vi "Valid data with Header (SubVI).vi"(10 "Header":string, 11 "Input data":string) -> (3 "Valid Data":string)   [LabVIEW 2021]
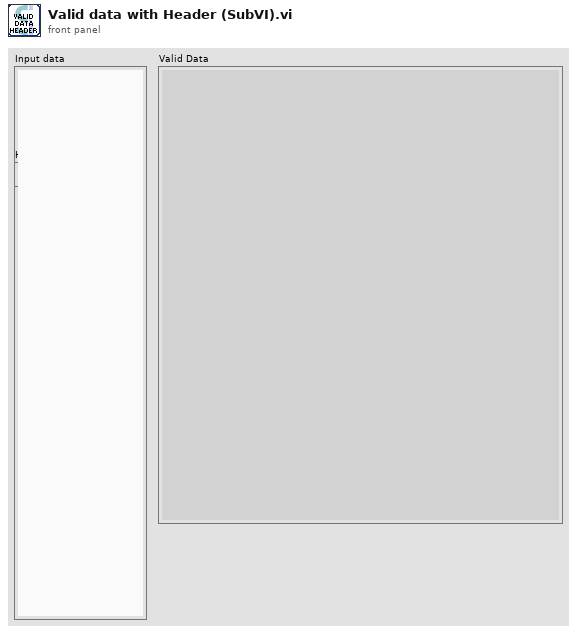
[diagram p1: front panel]
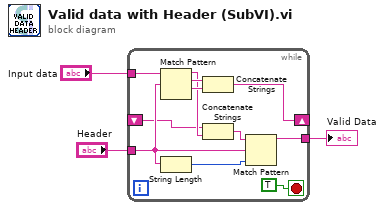
[diagram p0: block diagram]
diagram:
  n1 = while {
    tunnel: "Input data" -> [w11]
    tunnel: [w8] -> w2
    tunnel: "Header" -> [w7]
    shift-right: [w12] -> _
    shift-left: _ -> [w4]
    stop <- TRUE stop-if-true
    n2 = Match Pattern(string=w11, regular expression=w7) -> (before substring=w5:string, match substring=w14:string, after substring=w13:string)  [unwired: 1 in, 1 out]
    n3 = String Length(string=w7) -> (length=w9:i32)
    n4 = Concatenate Strings(w14, w13) -> (w12:string)
    n5 = Concatenate Strings(w4, w5) -> (w10:string)
    n6 = Match Pattern(string=w10, regular expression=w7, offset (0)=w9) -> (before substring=w8:string)  [unwired: 3 out]
  }
  "Valid Data" <- w2
